vi "fgvEventBack.vi"(8 "error in (no error)":errorcluster, 9 "Cmd":string, 10 "EventRefNum":refnum<event-registration>, 11 "EventData":refnum<user-event>) -> (0 "error out":errorcluster, 2 "EventRefNum out":refnum<event-registration>, 3 "EventData out":refnum<user-event>)   [LabVIEW 2013, in "CONTROLLER.lvclass"]
uses:
  CONTROLLER.lvclass
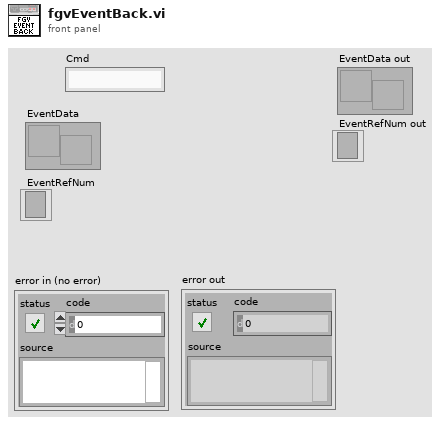
[diagram p1: front panel]
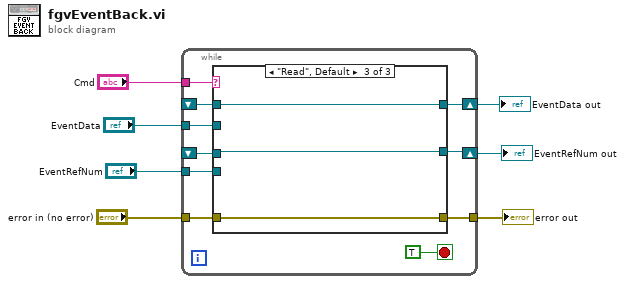
[diagram p0: block diagram]
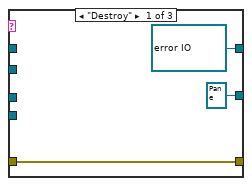
[diagram p2: hidden frame]
diagram:
  n1 = while {
    tunnel: "Cmd" -> [w16]
    shift-right: [w15] -> w1
    shift-left: _ -> [w10]
    tunnel: "EventData" -> [w14]
    shift-right: [w11] -> w2
    shift-left: _ -> [w13]
    tunnel: "EventRefNum" -> [w12]
    tunnel: "error in (no error)" -> [w9]
    tunnel: [w8] -> w5
    stop <- TRUE stop-if-true
    n2 = case shown="\"Read\", Default" w16 {
      tunnel: [refnum<user-event> refnum ("EventData") w23 w26] -> w15
      tunnel: w14 -> [_ w23 _]
      tunnel: w13 -> [_ _ w25]
      tunnel: [refnum<event-registration> refnum ("EventRefNum") w22 w25] -> w11
      tunnel: w12 -> [_ w22 _]
      tunnel: w10 -> [_ _ w26]
      tunnel: w9 -> [w20 w21 w24]
      tunnel: [w20 w21 w24] -> w8
      frame "Destroy" {
      }
      frame "Register" {
      }
      frame "Read", Default {
      }
    }
  }
  "error out" <- w5
  "EventData out" <- w1
  "EventRefNum out" <- w2
